vi "Test R_W.vi"() -> ()   [LabVIEW 2021]
uses:
  <vilib>/CIF Foundation/CIF Channels Core/CIF_NIChn/Double/CIF_NIChn_Double.lvclass
  <vilib>/CIF Foundation/CIF Channels Core/CIFChannels/Typedef/Direction.ctl
  <vilib>/CIF Foundation/CIF Channels Core/CIFChannels/CIFChannels.lvclass
  CIF-LVCore/src/CIFCore/Grpc/CIFCoreWrapper/CIFCoreWrapper.lvlib
  <vilib>/CIF Foundation/CIF Channels Core/CIF_NIChn/U64/CIF_NIChn_U64.lvclass
  CIF-LVCore/src/CIFCore/Grpc/CIFCoreChannel_client/RPC Messages/cif_channelcore_ConnectSubscriber.ctl
  CIF-LVCore/src/CIFCore/Grpc/CIFCoreChannel_client/CIFCoreChannel_client.lvlib
  CIF-LVCore/src/CIFCore/Common/Typedef/Plugin State.ctl
  CIF-LVCore/src/CIFCore/Common/CIFCoreCommon.lvlib
  CIF-LVCore/src/CIFCore/Common/Typedef/Timing Stats Base.ctl
  CIF-LVCore/src/CIFCore/Common/Typedef/Timing Statistics.ctl
  CIF-LVCore/src/CIFCore/Common/Typedef/FIFO Statistics.ctl
  CIF-LVCore/src/CIFCore/Common/Typedef/Simple Error.ctl
  CIF-LVCore/src/CIFCore/Common/Typedef/Monitor Doubles.ctl
  CIF-LVCore/src/CIFCore/Common/Typedef/Monitor U64.ctl
  CIF-LVCore/src/CIFCore/Common/Typedef/Monitor I64.ctl
  CIF-LVCore/src/CIFCore/Common/Typedef/gRPC Reported Plugin Status.ctl
panel:
  out "Data 4":u64
  out "error out 4":errorcluster
  out "Node Status":T1 {"Monitor Doubles"."4" format="%#_9g"; "Monitor Doubles"."3" format="%#_9g"; "Monitor Doubles"."2" format="%#_9g"; "Monitor Doubles"."1" format="%#_9g"}
  in  "address":string="192.168.1.160:50051"
  in  "Data 3":dbl
  out "error out 3":errorcluster
  in  "stop":bool
  out "error out":errorcluster
  out "Data 2":dbl
  in  "Data":dbl
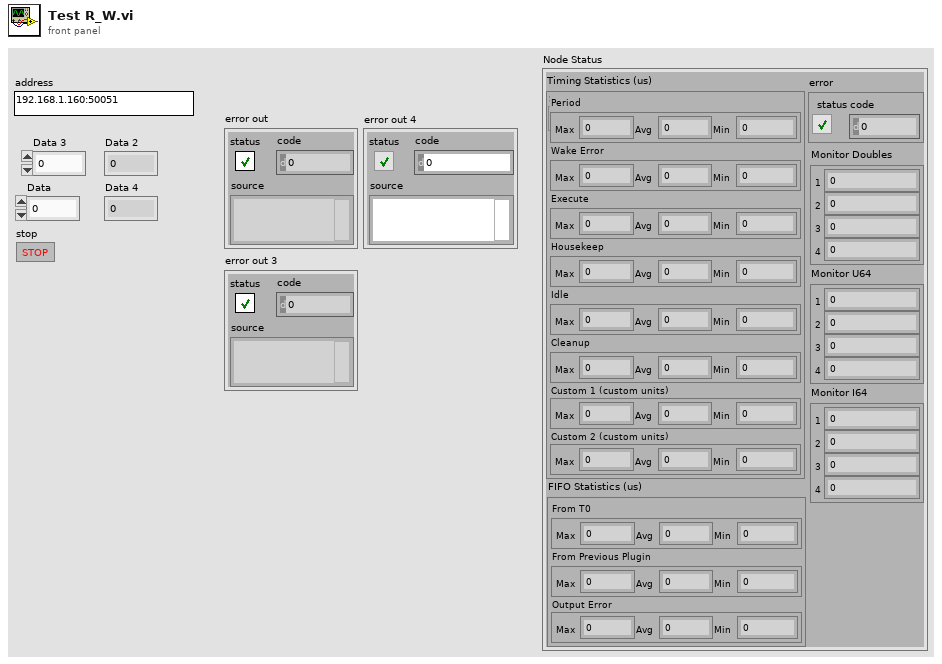
[diagram p1: front panel]
types:
  T1 = typedef "CIFCoreCommon.lvlib/gRPC Reported Plugin Status.ctl" = cluster{"State":T2, "Timing Statistics (us)":T3, "FIFO Statistics (us)":T5, "error":T6, "Monitor Doubles":T7, "Monitor U64":T8, "Monitor I64":T9}
  T2 = typedef "CIFCoreCommon.lvlib/Plugin State.ctl" = enum32{"Null", "Creating", "Listening", "Running", "CleaningUp", "Destroying"}
  T3 = typedef "CIFCoreCommon.lvlib/Timing Statistics.ctl" = cluster{"Period":T4, "Wake Error":T4, "Execute":T4, "Housekeep":T4, "Idle":T4, "Cleanup":T4, "Custom 1 (custom units)":T4, "Custom 2 (custom units)":T4}
  T4 = typedef "CIFCoreCommon.lvlib/Timing Stats Base.ctl" = cluster{"Max":i64, "Avg":dbl, "Min":i64}
  T5 = typedef "CIFCoreCommon.lvlib/FIFO Statistics.ctl" = cluster{"From T0":T4, "From Previous Plugin":T4, "Output Error":T4}
  T6 = typedef "CIFCoreCommon.lvlib/Simple Error.ctl" = cluster{"status":bool, "code":i32}
  T7 = typedef "CIFCoreCommon.lvlib/Monitor Doubles.ctl" = cluster{"1":dbl, "2":dbl, "3":dbl, "4":dbl}
  T8 = typedef "CIFCoreCommon.lvlib/Monitor U64.ctl" = cluster{"1":u64, "2":u64, "3":u64, "4":u64}
  T9 = typedef "CIFCoreCommon.lvlib/Monitor I64.ctl" = cluster{"1":i64, "2":i64, "3":i64, "4":i64}
  T10 = typedef "CIFCoreChannel_client.lvlib/cif_channelcore_ConnectSubscriber.ctl" = cluster{"subscriber_name":string, "publisher_name":string, "custom_connect":u8[]}
  T11 = typedef "CIFChannels.lvclass/Direction.ctl" = enum16{"Publisher", "Subscriber"}
  T12 = typedef "grpc-lvsupport-release.lvlib/grpcId.ctl" = u64
  T13 = typedef "CIFCoreChannel_client.lvlib/cif_channelcore_Channel.ctl" = cluster{"name":string, "direction":T14, "type":string, "custom_config":u8[], "connected":bool, "connected_name":string, "forced":bool, "multi_writer":bool}
  T14 = typedef "CIFCoreChannel_client.lvlib/cif_channelcore_Direction.ctl" = enum32{"PUBLISHER", "SUBSCRIBER"}
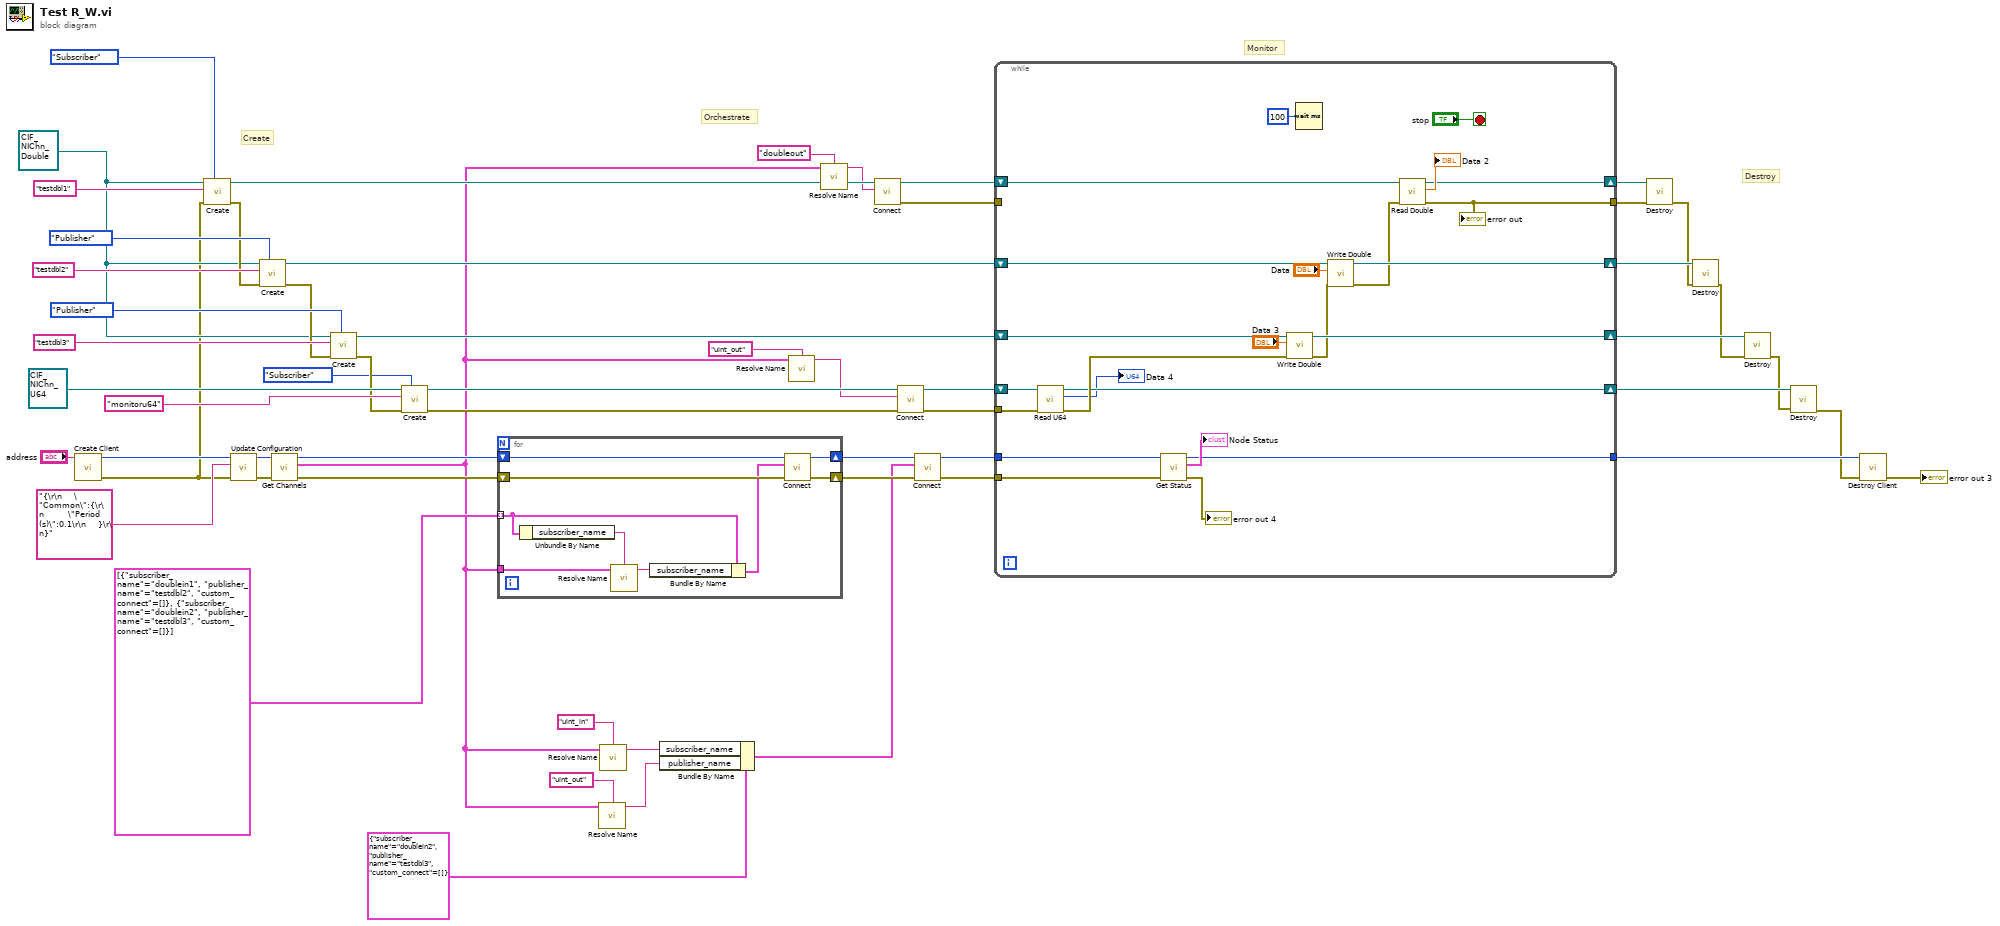
[diagram p0: block diagram]
diagram:
  w41 = refnum<class "CIF_NIChn_Double.lvclass"> refnum ("CIFTag in")
  # "Destroy"
  # "Monitor"
  # "Orchestrate"
  # "Create"
  n1 = call "Create Client.vi"("address"="address") -> ("error out"=w22:errorcluster, "gRPC ID Out"=w23:T12)  [unwired: 9 in]
  n2 = call-dynamic "Create.vi"("Direction"=Direction."Subscriber", "error in (no error)"=w22, "Name"="testdbl1", "CIFTag in"=w41) -> ("error out"=w52:errorcluster, "CIFTag out"=w38:refnum<class "CIF_NIChn_Double.lvclass">)  [unwired: 6 in]
  n3 = call "Update Configuration.vi"("error in"=w22, "JSON Configuration"="{\r\n    \"Common\":{\r\n        \"Period (s)\":0.1\r\n    }\r\n}" ("JSON Configuration in"), "gRPC ID"=w23) -> ("error out"=w20:errorcluster, "gRPC ID out"=w21:T12)  [unwired: 7 in]
  n4 = call-dynamic "Create.vi"("Direction"=Direction."Publisher", "error in (no error)"=w52, "Name"="testdbl2", "CIFTag in"=w41) -> ("error out"=w43:errorcluster, "CIFTag out"=w55:refnum<class "CIF_NIChn_Double.lvclass">)  [unwired: 6 in]
  n5 = call "Get Channels.vi"("error in"=w20, "gRPC ID"=w21) -> ("error out"=w19:errorcluster, "Channels"=w1:T13[], "gRPC ID out"=w18:T12)  [unwired: 7 in]
  n6 = call-dynamic "Create.vi"("Direction"=Direction."Publisher", "error in (no error)"=w43, "Name"="testdbl3", "CIFTag in"=w41) -> ("error out"=w32:errorcluster, "CIFTag out"=w45:refnum<class "CIF_NIChn_Double.lvclass">)  [unwired: 6 in]
  n7 = call-dynamic "Create.vi"("Direction"=Direction."Subscriber", "error in (no error)"=w32, "Name"="monitoru64", "CIFTag in"=refnum<class "CIF_NIChn_U64.lvclass"> refnum) -> ("error out"=w29:errorcluster, "CIFTag out"=w31:refnum<class "CIF_NIChn_U64.lvclass">)  [unwired: 6 in]
  n8 = for {
    tunnel: T10[] [{"subscriber_name"="doublein1", "publisher_name"="testdbl2", "custom_connect"=[]}, {"subscriber_name"="doublein2", "publisher_name"="testdbl3", "custom_connect"=[]}] -> [w61] mode=indexing
    shift-right: [w64] -> w6
    shift-left: w19 -> [w65]
    shift-right: [w63] -> w7
    shift-left: w18 -> [w66]
    tunnel: w1 -> [w58]
    n9 = Unbundle By Name(w61) -> ("subscriber_name"=w62:string)
    n10 = call "Resolve Name.vi"("Channels"=w58, "Name"=w62) -> ("Resolved Name"=w60:string)  [unwired: 2 in]
    n11 = Bundle By Name(cluster=w61, "subscriber_name"=w60) -> (w59:T10)
    n12 = call "Connect.vi"("error in"=w65, "Connection"=w59, "gRPC ID"=w66) -> ("error out"=w64:errorcluster, "gRPC ID out"=w63:T12)  [unwired: 7 in]
  }
  n13 = call "Resolve Name.vi"("Channels"=w1, "Name"="uint_out") -> ("Resolved Name"=w8:string)  [unwired: 2 in]
  n14 = call "Resolve Name.vi"("Channels"=w1, "Name"="uint_in") -> ("Resolved Name"=w9:string)  [unwired: 2 in]
  n15 = Bundle By Name(cluster=T10 {"subscriber_name"="doublein2", "publisher_name"="testdbl3", "custom_connect"=[]} ("Connection"), "subscriber_name"=w9, "publisher_name"=w8) -> (w3:T10)
  n16 = call "Resolve Name.vi"("Channels"=w1, "Name"="uint_out" ("Connection Name")) -> ("Resolved Name"=w16:string)  [unwired: 2 in]
  n17 = call "Resolve Name.vi"("Channels"=w1, "Name"="doubleout" ("Connection Name")) -> ("Resolved Name"=w15:string)  [unwired: 2 in]
  n18 = call-dynamic "Connect.vi"("Connection Name"=w15, "CIFTag in"=w38) -> ("error out"=w2:errorcluster, "CIFTag out"=w37:refnum<class "CIF_NIChn_Double.lvclass">)  [unwired: 8 in]
  n19 = call-dynamic "Connect.vi"("error in (no error)"=w29, "Connection Name"=w16, "CIFTag in"=w31) -> ("error out"=w28:errorcluster, "CIFTag out"=w30:refnum<class "CIF_NIChn_U64.lvclass">)  [unwired: 7 in]
  n20 = call "Connect.vi"("error in"=w6, "Connection"=w3, "gRPC ID"=w7) -> ("error out"=w4:errorcluster, "gRPC ID out"=w5:T12)  [unwired: 7 in]
  n21 = while {
    shift-right: [w87] -> w51
    shift-left: w37 -> [w77]
    shift-right: [w86] -> w50
    shift-left: w55 -> [w90]
    tunnel: [w84] -> w49
    shift-right: [w81] -> w47
    shift-left: w45 -> [w79]
    tunnel: w5 -> [w75]
    tunnel: w4 -> [w74]
    tunnel: [w72] -> w36
    tunnel: w28 -> [w70]
    shift-right: [w68] -> w27
    shift-left: w30 -> [w71]
    tunnel: w2 -> [_]
    stop <- "stop" stop-if-true
    n22 = call-dynamic "Read U64.vi"("error in (no error)"=w70, "CIFTag in"=w71) -> ("error out"=w69:errorcluster, "Data"=→"Data 4":u64, "CIFTag out"=w68:refnum<class "CIF_NIChn_U64.lvclass">)  [unwired: 6 in, 1 out]
    n23 = call "Get Status.vi"("error in"=w74, "gRPC ID"=w75) -> ("error out"=→"error out 4":errorcluster, "Node Status"=→"Node Status":T1, "gRPC ID out"=w72:T12)  [unwired: 7 in]
    n24 = call-dynamic "Write Double.vi"("error in (no error)"=w69, "Data"="Data 3", "CIFTag in"=w79) -> ("error out"=w78:errorcluster, "CIFTag out"=w81:refnum<class "CIF_NIChn_Double.lvclass">)  [unwired: 6 in, 1 out]
    n25 = Wait (ms)(milliseconds to wait=u32 100) -> ()  [unwired: 1 out]
    n26 = call-dynamic "Write Double.vi"("error in (no error)"=w78, "Data"="Data", "CIFTag in"=w90) -> ("error out"=w85:errorcluster, "CIFTag out"=w86:refnum<class "CIF_NIChn_Double.lvclass">)  [unwired: 6 in, 1 out]
    n27 = call-dynamic "Read Double.vi"("error in (no error)"=w85, "CIFTag in"=w77) -> ("error out"=w84:errorcluster, "Data"=→"Data 2":dbl, "CIFTag out"=w87:refnum<class "CIF_NIChn_Double.lvclass">)  [unwired: 6 in, 1 out]
    "error out" <- w84
  }
  n28 = call-dynamic "Destroy.vi"("error in (no error)"=w49, "CIFTag in"=w51) -> ("error out"=w48:errorcluster)  [unwired: 8 in, 1 out]
  n29 = call-dynamic "Destroy.vi"("error in (no error)"=w48, "CIFTag in"=w50) -> ("error out"=w42:errorcluster)  [unwired: 8 in, 1 out]
  n30 = call-dynamic "Destroy.vi"("error in (no error)"=w42, "CIFTag in"=w47) -> ("error out"=w26:errorcluster)  [unwired: 8 in, 1 out]
  n31 = call-dynamic "Destroy.vi"("error in (no error)"=w26, "CIFTag in"=w27) -> ("error out"=w25:errorcluster)  [unwired: 8 in, 1 out]
  n32 = call "Destroy Client.vi"("error in"=w25, "gRPC ID"=w36) -> ("error out"=→"error out 3":errorcluster)  [unwired: 9 in]
